vi "arrayMatrixVI.vi"() -> ()   [LabVIEW 2012]
uses:
  <vilib>/Analysis/Matrix/Datatypes/RealMatrix.ctl
  <vilib>/Analysis/Matrix/Numeric/Conversions/Array To Matrix - RA2.vi
  <vilib>/Analysis/Matrix/NI_Matrix.lvlib
panel:
  out "Real Matrix":T1
  out "size(s)":i32[](array[numeric])
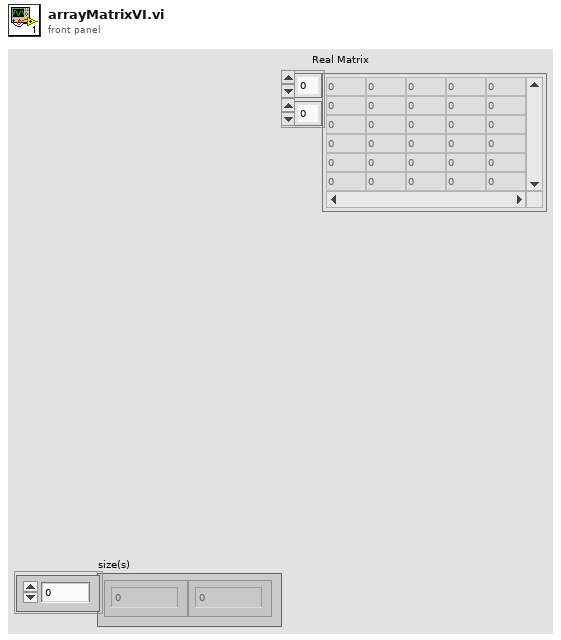
[diagram p1: front panel]
types:
  T1 = typedef "NI_Matrix.lvlib/RealMatrix.ctl" = dbl[][]
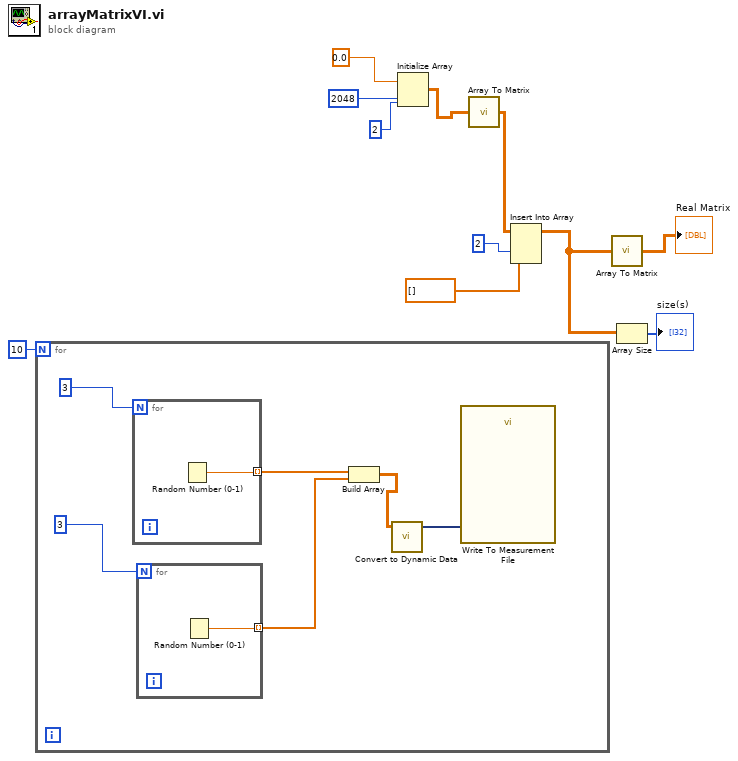
[diagram p0: block diagram]
diagram:
  n1 = for {
    N: 10 -> [_]
    n2 = for {
      N: 3 -> [_]
      tunnel: [w18] -> w14 mode=indexing
      n3 = Random Number (0-1)() -> (number: 0 to 1=w18:dbl)
    }
    n4 = for {
      N: 3 ("Numeric Control") -> [_]
      tunnel: [w19] -> w15 mode=indexing
      n5 = Random Number (0-1)() -> (number: 0 to 1=w19:dbl)
    }
    n6 = Build Array(w14, w15) -> (w12:T1)
    n7 = call "Convert to Dynamic Data"("2D Array"=w12) -> ("Dynamic Data Type"=w13:dynamicdata)  [unwired: 3 in]
    n8 = call "Write To Measurement File"("Signals"=w13) -> ()  [unwired: 16 in, 3 out]
  }
  n9 = Initialize Array(0.0 ("element"), 2048 ("dimension size"), 2 ("dimension size")) -> (w6:dbl[][])
  n10 = call-poly <vilib>:"Array To Matrix.vi"("Real 2D Array"=w6) -> ("Real Matrix"=w3:T1)
  n11 = Insert Into Array(array=w3, index (col)=2 ("disabled index (col)"), new element=dbl[] [] ("new element/subarray")) -> (w5:T1)  [unwired: 1 in]
  n12 = call-poly <vilib>:"Array To Matrix.vi"("Real 2D Array"=w5) -> ("Real Matrix"=→"Real Matrix":T1)
  n13 = Array Size(array=w5) -> (size(s)=→"size(s)":i32[])
